vi "Hydrosonic_Conrol.vi"(2 "In range %":dbl format="%.2f", 3 "Input Mode":enum16{"Desired Frequency", "Transducer value"}(ring), 4 "Actual Sampling rate (Hz)":dbl=1000.0 format="%.2f", 5 "Desired Value":dbl format="%.2f") -> (0 "Error Info":string, 1 "Set output":dbl format="%.2f")   [LabVIEW 2010]
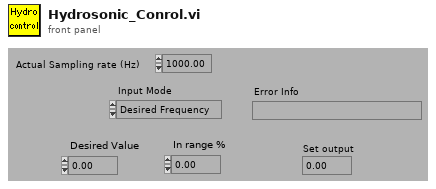
[diagram p1: front panel]
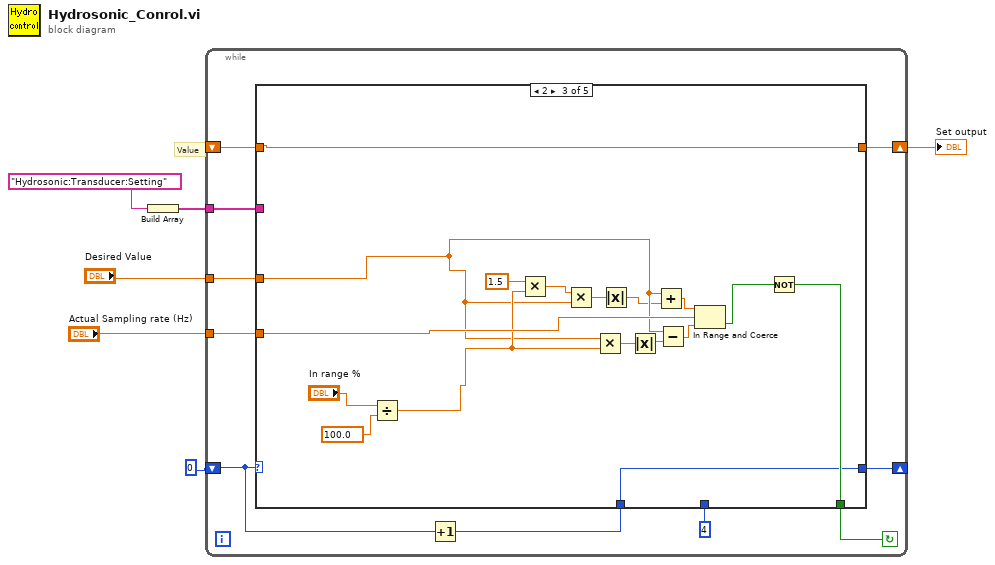
[diagram p0: block diagram]
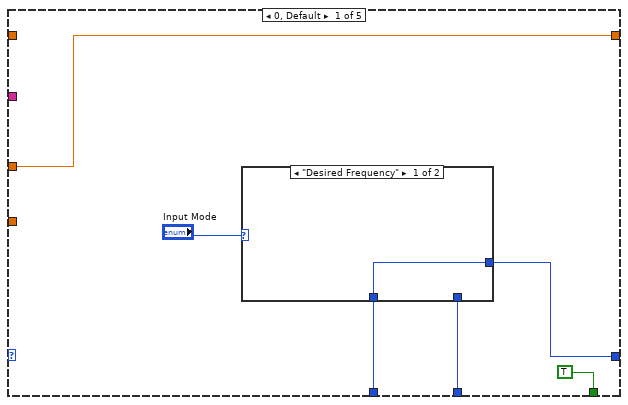
[diagram p2: hidden frame]
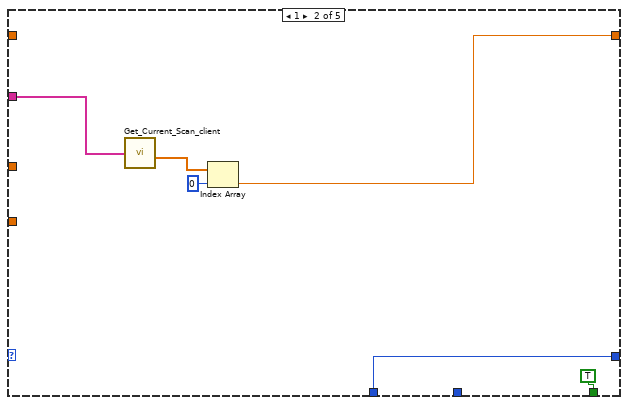
[diagram p4: hidden frame]
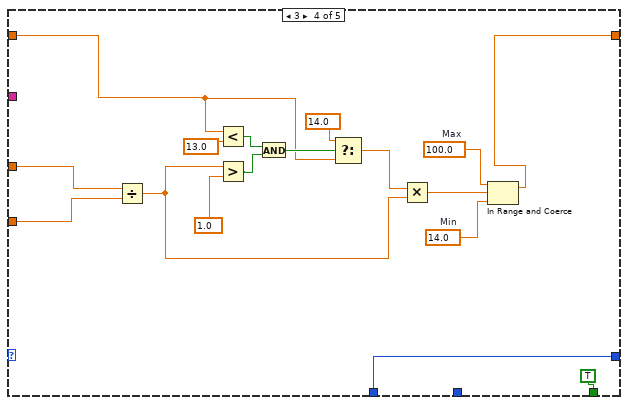
[diagram p5: hidden frame]
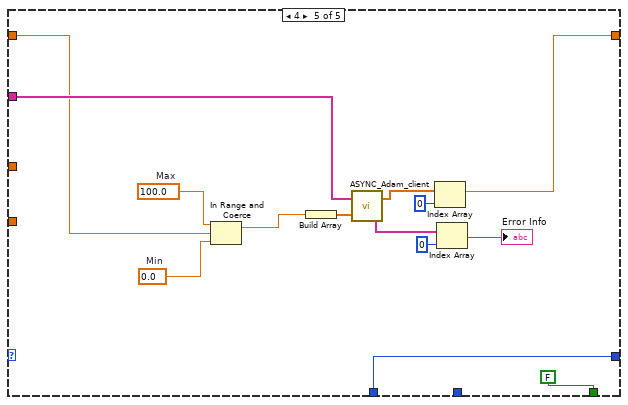
[diagram p6: hidden frame]
diagram:
  # "Value"
  n1 = Build Array("Hydrosonic:Transducer:Setting") -> (w3:string[])
  n2 = while {
    tunnel: "Actual Sampling rate (Hz)" -> [w9]
    tunnel: w3 -> [w11]
    shift-left: _ -> [w8]
    shift-right: [w10] -> w1
    tunnel: "Desired Value" -> [w16]
    shift-left: 0 -> [w15]
    shift-right: [w14] -> _
    stop <- w12 continue-if-true
    n3 = Increment(x=w15) -> (x+1=w13:i32)
    n4 = case shown="2" w15 {
      tunnel: w16 -> [w18 _ w33 w62 _]
      tunnel: [w21 w26 w46 w64 w77] -> w14
      tunnel: w13 -> [w20 w26 w46 w64 w77]
      tunnel: [TRUE TRUE w47 TRUE FALSE] -> w12
      tunnel: w11 -> [_ w30 _ _ w69]
      tunnel: [w18 w27 w45 w48 w65] -> w10
      tunnel: w9 -> [_ _ w41 w61 _]
      tunnel: w8 -> [_ _ w45 w54 w67]
      tunnel: 4 -> [w17 _ _ _ _]
      frame 0, Default {
        n5 = case shown="\"Desired Frequency\"" "Input Mode" {
          tunnel: [w23 w24] -> w21
          tunnel: w20 -> [w23 _]
          tunnel: w17 -> [_ w24]
          frame "Desired Frequency" {
          }
          frame "Transducer value" {
          }
        }
      }
      frame 1 {
        n6 = call "Get_Current_Scan_client.vi"("ADAM Ch Names"=w30) -> ("Numerical Values"=w29:dbl[])  [unwired: 3 out]
        n7 = Index Array(array=w29, index=0 ("Index")) -> (element=w27:dbl)
      }
      frame 2 {
        n8 = Divide(x="In range %", y=100.0) -> (x/y=w36:dbl)
        n9 = Multiply(x=1.5, y=w36) -> (x*y=w34:dbl)
        n10 = Multiply(x=w34, y=w33) -> (x*y=w35:dbl)
        n11 = Multiply(x=w33, y=w36) -> (x*y=w42:dbl)
        n12 = Absolute Value(x=w35) -> (abs(x)=w32:dbl)
        n13 = Absolute Value(x=w42) -> (abs(x)=w38:dbl)
        n14 = Add(x=w33, y=w32) -> (x+y=w44:dbl)
        n15 = Subtract(x=w33, y=w38) -> (x-y=w43:dbl)
        n16 = In Range and Coerce(upper limit=w44, x=w41, lower limit=w43) -> (In Range?=w31:bool)  [unwired: 1 out]
        n17 = Not(x=w31) -> (.not. x?=w47:bool)
      }
      frame 3 {
        w50 = 100.0  # Max
        w51 = 14.0  # Min
        n18 = Divide(x=w62, y=w61) -> (x/y=w52:dbl)
        n19 = Less?(x=w54, y=13.0) -> (x < y?=w57:bool)
        n20 = Greater?(x=w52, y=1.0) -> (0:w58:bool)
        n21 = And(x=w57, y=w58) -> (x .and. y?=w56:bool)
        n22 = Select(t=14.0, s=w56, f=w54) -> (s? t:f=w53:dbl)
        n23 = Multiply(x=w53, y=w52) -> (x*y=w49:dbl)
        n24 = In Range and Coerce(upper limit=w50, x=w49, lower limit=w51) -> (coerced(x)=w48:dbl)  [unwired: 1 out]
      }
      frame 4 {
        w75 = 100.0  # Max
        w76 = 0.0  # Min
        n25 = In Range and Coerce(upper limit=w75, x=w67, lower limit=w76) -> (coerced(x)=w66:dbl)  [unwired: 1 out]
        n26 = Build Array(w66) -> (w72:dbl[])
        n27 = call "ASYNC_Adam_client.vi"("Values"=w72, "Channel Names"=w69) -> ("Scan Comments"=w70:string[], "Calibrated Units"=w71:dbl[])
        n28 = Index Array(array=w71, index=0 ("Index")) -> (element=w65:dbl)
        n29 = Index Array(array=w70, index=0 ("Index")) -> (element=→"Error Info":string)
      }
    }
  }
  "Set output" <- w1
